vi "SRV_Motor Control Buttons Template.vi"() -> ()   [LabVIEW 2009]
uses:
  SRV VIs/Motors/Motors Config/SRV_Motor Control Button Icons_TRUE.ctl
  SRV VIs/Motors/Motors Config/SRV_Motor Control Button Icons_FALSE.ctl
panel:
  in  "button 10":bool
  out "true 10":T1
  out "false 10":T2
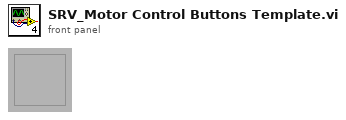
[diagram p1: front panel]
types:
  T1 = typedef "SRV_Motor Control Button Icons_TRUE.ctl" = u16
  T2 = typedef "SRV_Motor Control Button Icons_FALSE.ctl" = u16
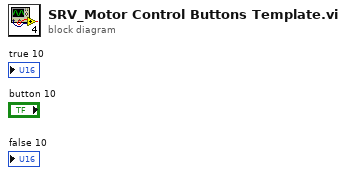
[diagram p0: block diagram]
diagram:
